vi "RemoveAt.vi"(8 "error in (no error)":errorcluster caption="错误输入（无错误）", 10 "index":i32, 11 "ArrayListClass 输入":refnum<class "ArrayListClass.lvclass"> caption="DNL_LabVIEW Object in") -> (0 "error out":errorcluster caption="错误输出", 3 "ArrayListClass 输出":refnum<class "ArrayListClass.lvclass"> caption="DNL_LabVIEW Object out")   [LabVIEW 2012, in "ArrayListClass.lvclass"]
uses:
  ArrayListClass.lvclass
  ArrayListClass.lvclass/ArrayListClass.ctl
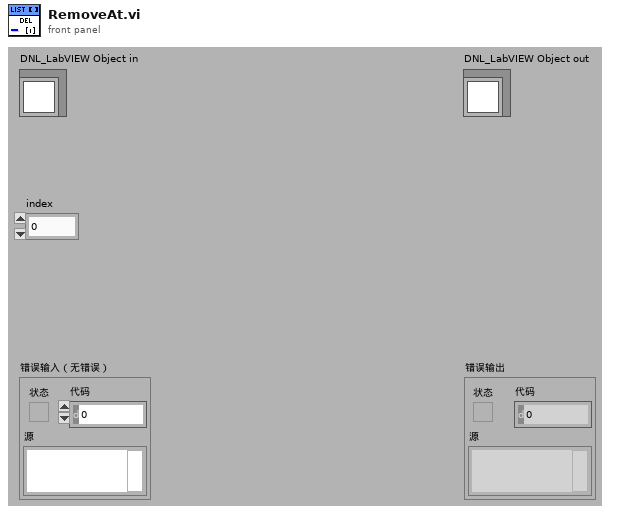
[diagram p1: front panel]
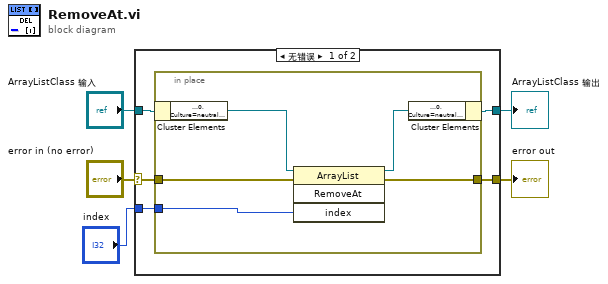
[diagram p0: block diagram]
diagram:
  n1 = case shown="无错误" "error in (no error)" {
    selector: "error in (no error)" -> [w8 w17]
    tunnel: [w7 w17] -> w4
    tunnel: [w9 w16] -> w2
    tunnel: "ArrayListClass 输入" -> [w10 w16]
    tunnel: "index" -> [w6 _]
    frame No Error {
      n2 = in-place {
        in-place-border: w8 -> [w13]
        in-place-border: [w12] -> w7
        in-place-border: w6 -> [w11]
        n3 = in-place-cluster #1(w10) -> ("ArrayList"=w15:refnum<k24>)
        n4 = invoke class="ArrayList" method="RemoveAt"(reference=w15, error in=w13, "index"=w11) -> (reference out=w14:refnum<k24>, error out=w12:errorcluster)  [unwired: 1 in, 2 out]
        n5 = in-place-cluster #1("ArrayList"=w14) -> (w9:refnum<class "ArrayListClass.lvclass">)
      }
    }
    frame Error {
    }
  }
  "error out" <- w4
  "ArrayListClass 输出" <- w2
